vi "Step Association Get By Station.vi"(8 "error in (no error)":errorcluster, 10 "iStation (0)":i32, 11 "Connection Refnum":T2) -> (0 "error out":errorcluster, 2 "Step Associations":T1[](array[typedef]), 3 "Connection Refnum":T2, 4 "Data Present?":bool)   [LabVIEW 2011]
uses:
  SI.LIB/ODBC/SQL Controls/Connection Refnum.ctl
  Step Association Record.ctl
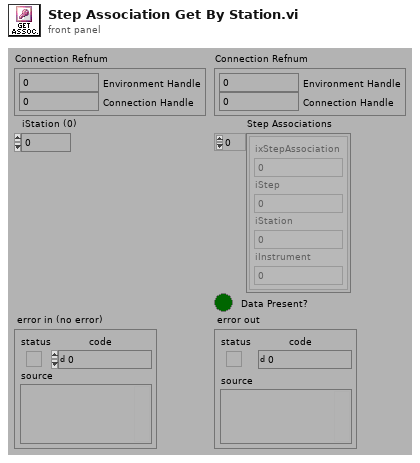
[diagram p1: front panel]
types:
  T1 = typedef "Step Association Record.ctl" = cluster{"ixStepAssociation":i32, "iStep":i32, "iStation":i32, "iInstrument":i32}
  T2 = typedef "Connection Refnum.ctl" = cluster{"Environment Handle":i32, "Connection Handle":i32}
  T3 = typedef "Statement Refnum.ctl" = cluster{"Statement Handle":i32, "Parameter Number":u16}
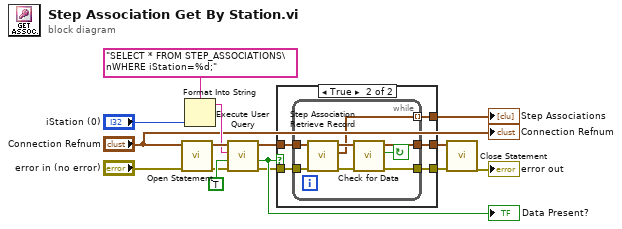
[diagram p0: block diagram]
diagram:
  n1 = call "Open Statement.vi"("error in (no error)"="error in (no error)", "Connection Refnum"="Connection Refnum") -> ("error out"=w7:errorcluster, "Statement Refnum"=w8:T3)  [unwired: 4 out]
  n2 = Format Into String(format string="SELECT * FROM STEP_ASSOCIATIONS\nWHERE iStation=%d;" ("User Query"), "iStation (0)") -> (resulting string=w6:string)  [unwired: 2 in, 1 out]
  n3 = call "Execute User Query.vi"("error in (no error)"=w7, "Return Data? (f)"=TRUE, "User Query"=w6, "Statement Refnum"=w8) -> ("error out"=w14:errorcluster, "Data Present?"=w15:bool, "Statement Refnum"=w13:T3)  [unwired: 1 out]
  "Data Present?" <- w15
  n4 = case shown="True" w15 {
    tunnel: w14 -> [w16 w22]
    tunnel: w13 -> [w17 w21]
    tunnel: [w16 w20] -> w10
    tunnel: [w17 w19] -> w11
    tunnel: [_ w18] -> w3
    frame False {
    }
    frame True {
      n5 = while {
        tunnel: w22 -> [w30]
        tunnel: w21 -> [w29]
        tunnel: [w23] -> w18 mode=indexing
        tunnel: [w26] -> w20
        tunnel: [w25] -> w19
        stop <- w24 continue-if-true
        n6 = call "Step Association Retrieve Record.vi"("error in (no error)"=w30, "Statement Refnum"=w29) -> ("error out"=w27:errorcluster, "Association"=w23:T1, "Statement Refnum"=w28:T3)  [unwired: 7 in]
        n7 = call "Check for Data.vi"("error in (no error)"=w27, "Statement Refnum"=w28) -> ("error out"=w26:errorcluster, "Data Present?"=w24:bool, "Statement Refnum"=w25:T3)  [unwired: 3 out]
      }
    }
  }
  "Step Associations" <- w3
  n8 = call "Close Statement.vi"("error in (no error)"=w10, "Statement Refnum"=w11) -> ("error out"=→"error out":errorcluster)  [unwired: 5 out]
  "Connection Refnum" <- "Connection Refnum"
